vi "test Next Frame Check.vi"(8 "error in (no error)":errorcluster, 11 "BC Major Frame in":refnum<class "BC Major Frame.lvclass">) -> (0 "error out":errorcluster, 3 "BC Major Frame out":refnum<class "BC Major Frame.lvclass">)   [LabVIEW 2016, in "BC Major Frame.lvclass"]
uses:
  BC Major Frame.lvclass
  Frames & Messages/TypeDefs/BC Condition Codes.ctl
  Frames & Messages/TypeDefs/BC Op Codes - Verbose.ctl
  PPLs/FPGA Interface.lvlibp/FPGA Interface/FPGA Interface.lvclass
  BCI-1553 API.lvlib
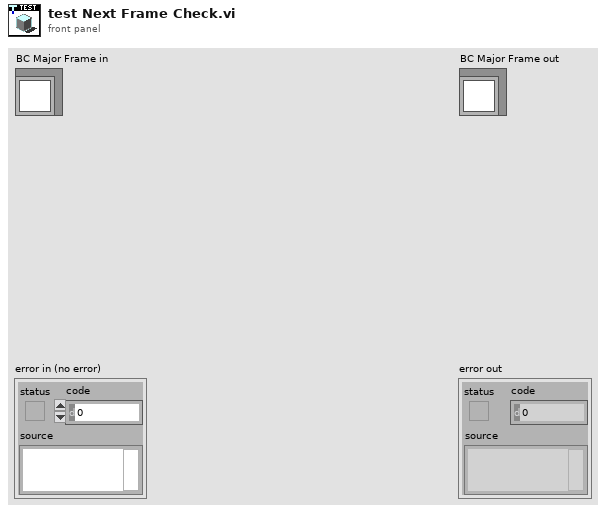
[diagram p1: front panel]
types:
  T1 = typedef "BCI-1553 API.lvlib/BC Op Codes - Verbose.ctl" = enum16{"EXECUTE MSG", "EXECUTE MSG GO", "JUMP", "CALL SUBROUTINE", "RETURN", "INTERRUPT REQUEST", "HALT", "DELAY", "WAIT FRAME TIMER = 0", "COMPARE FRAME TIMER", "COMPARE MSG TIMER", "LOAD TIME TAG CTR", "LOAD TIME TAG CTR HI", "LOAD FRAME TIMER", "START FRAME TIMER", "PUSH TIME TAG COUNT", "PUSH TIME TAG COUNT HI", "PUSH TIME TAG COUNT BOTH", "PUSH BLOCK STATUS WORD", "PUSH CURRENT VALUE", "PUSH INDIRECT", "WAIT EXT TRIGGER", "EXECUTE AND FLIP", "EXECUTE, FLIP, GO", "WRITE VALUE TO WMI", "WRITE VALUE TO MEM", "DECREMENT RAM, SKIP", "FLAG"}
  T2 = typedef "BCI-1553 API.lvlib/BC Condition Codes.ctl" = enum16{"GP0 == 1 || LT", "GP1 == 1 || NE", "GP2 == 1", "GP3 == 1", "GP4 == 1", "GP5 == 1", "GP6 == 1", "GP7 == 1", "NORESP", "FMTERR", "GOODBLOCK", "MSKSTATSET", "BADMSG", "1RETRY", "2RETRY", "ALWAYS"}
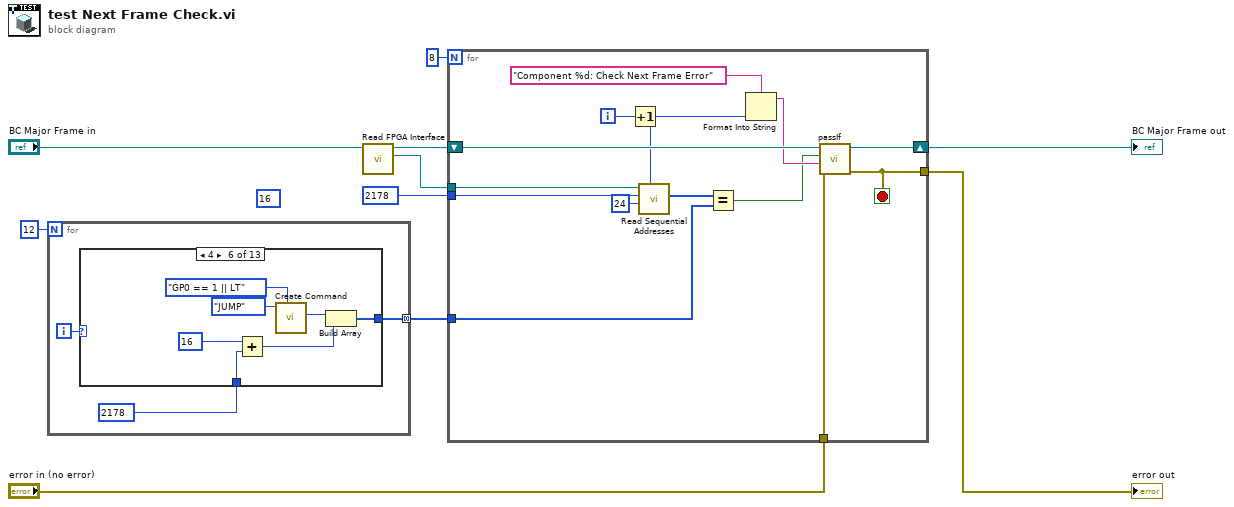
[diagram p0: block diagram]
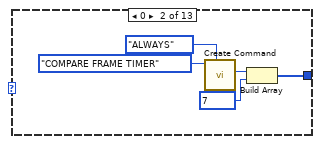
[diagram p3: hidden frame]
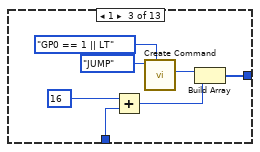
[diagram p4: hidden frame]
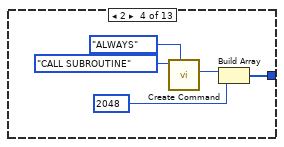
[diagram p5: hidden frame]
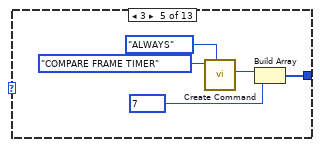
[diagram p6: hidden frame]
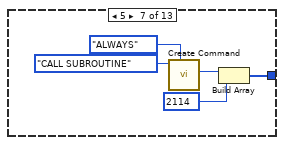
[diagram p7: hidden frame]
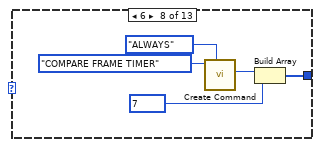
[diagram p8: hidden frame]
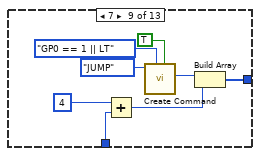
[diagram p9: hidden frame]
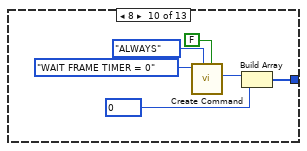
[diagram p10: hidden frame]
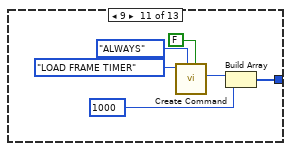
[diagram p11: hidden frame]
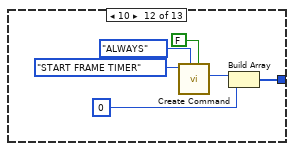
[diagram p12: hidden frame]
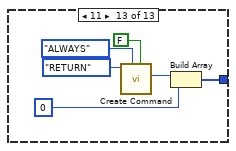
[diagram p13: hidden frame]
diagram:
  (unwired) u16 16 ("element")
  n1 = for {
    N: 12 -> [_]
    tunnel: [w12] -> w1 mode=concatenating
    i -> [w13]
    n2 = case shown="4" w13 {
      tunnel: [_ w15 w22 w27 w32 w39 w44 w49 w57 w63 w69 w75 w81] -> w12
      tunnel: u16 2178 -> [_ _ w19 _ _ w36 _ _ w53 _ _ _ _]
      frame Default {
      }
      frame 0 {
        n3 = call "Create Command.vi"("Condition"=BC_Condition_Codes."ALWAYS", "Op Code"=BC_Op_Codes_-_Verbose."COMPARE FRAME TIMER") -> ("Instruction"=w16:u16)  [unwired: 8 in, 1 out]
        n4 = Build Array(w16, u16 7 ("element")) -> (w15:u16[])
      }
      frame 1 {
        n5 = Add(x=u16 16 ("element"), y=w19) -> (x+y=w21:u16)
        n6 = call "Create Command.vi"("Condition"=BC_Condition_Codes."GP0 == 1 || LT", "Op Code"=BC_Op_Codes_-_Verbose."JUMP") -> ("Instruction"=w23:u16)  [unwired: 8 in, 1 out]
        n7 = Build Array(w23, w21) -> (w22:u16[])
      }
      frame 2 {
        n8 = call "Create Command.vi"("Condition"=BC_Condition_Codes."ALWAYS", "Op Code"=BC_Op_Codes_-_Verbose."CALL SUBROUTINE") -> ("Instruction"=w28:u16)  [unwired: 8 in, 1 out]
        n9 = Build Array(w28, u16 2048) -> (w27:u16[])
      }
      frame 3 {
        n10 = call "Create Command.vi"("Condition"=BC_Condition_Codes."ALWAYS", "Op Code"=BC_Op_Codes_-_Verbose."COMPARE FRAME TIMER") -> ("Instruction"=w33:u16)  [unwired: 8 in, 1 out]
        n11 = Build Array(w33, u16 7) -> (w32:u16[])
      }
      frame 4 {
        n12 = Add(x=u16 16 ("element"), y=w36) -> (x+y=w37:u16)
        n13 = call "Create Command.vi"("Condition"=BC_Condition_Codes."GP0 == 1 || LT", "Op Code"=BC_Op_Codes_-_Verbose."JUMP") -> ("Instruction"=w40:u16)  [unwired: 8 in, 1 out]
        n14 = Build Array(w40, w37) -> (w39:u16[])
      }
      frame 5 {
        n15 = call "Create Command.vi"("Condition"=BC_Condition_Codes."ALWAYS", "Op Code"=BC_Op_Codes_-_Verbose."CALL SUBROUTINE") -> ("Instruction"=w45:u16)  [unwired: 8 in, 1 out]
        n16 = Build Array(w45, u16 2114) -> (w44:u16[])
      }
      frame 6 {
        n17 = call "Create Command.vi"("Condition"=BC_Condition_Codes."ALWAYS", "Op Code"=BC_Op_Codes_-_Verbose."COMPARE FRAME TIMER") -> ("Instruction"=w50:u16)  [unwired: 8 in, 1 out]
        n18 = Build Array(w50, u16 7) -> (w49:u16[])
      }
      frame 7 {
        n19 = Add(x=u16 4 ("element"), y=w53) -> (x+y=w55:u16)
        n20 = call "Create Command.vi"("Invert Condition (F)"=TRUE, "Condition"=BC_Condition_Codes."GP0 == 1 || LT", "Op Code"=BC_Op_Codes_-_Verbose."JUMP") -> ("Instruction"=w58:u16)  [unwired: 7 in, 1 out]
        n21 = Build Array(w58, w55) -> (w57:u16[])
      }
      frame 8 {
        n22 = call "Create Command.vi"("Invert Condition (F)"=FALSE, "Condition"=BC_Condition_Codes."ALWAYS", "Op Code"=BC_Op_Codes_-_Verbose."WAIT FRAME TIMER = 0") -> ("Instruction"=w64:u16)  [unwired: 7 in, 1 out]
        n23 = Build Array(w64, u16 0) -> (w63:u16[])
      }
      frame 9 {
        n24 = call "Create Command.vi"("Invert Condition (F)"=FALSE, "Condition"=BC_Condition_Codes."ALWAYS", "Op Code"=BC_Op_Codes_-_Verbose."LOAD FRAME TIMER") -> ("Instruction"=w70:u16)  [unwired: 7 in, 1 out]
        n25 = Build Array(w70, u16 1000) -> (w69:u16[])
      }
      frame 10 {
        n26 = call "Create Command.vi"("Invert Condition (F)"=FALSE, "Condition"=BC_Condition_Codes."ALWAYS", "Op Code"=BC_Op_Codes_-_Verbose."START FRAME TIMER") -> ("Instruction"=w76:u16)  [unwired: 7 in, 1 out]
        n27 = Build Array(w76, u16 0) -> (w75:u16[])
      }
      frame 11 {
        n28 = call "Create Command.vi"("Invert Condition (F)"=FALSE, "Condition"=BC_Condition_Codes."ALWAYS", "Op Code"=BC_Op_Codes_-_Verbose."RETURN") -> ("Instruction"=w82:u16)  [unwired: 7 in, 1 out]
        n29 = Build Array(w82, u16 0) -> (w81:u16[])
      }
    }
  }
  n30 = call-dynamic "Read FPGA Interface.vi"("1553 Test in"="BC Major Frame in") -> ("FPGA Interface"=w9:refnum<class "FPGA Interface.lvclass">, "1553 Test out"=w10:refnum<class "BC Major Frame.lvclass">)  [unwired: 8 in, 1 out]
  n31 = for {
    N: 8 -> [_]
    shift-right: [w98] -> w5
    shift-left: w10 -> [w97]
    tunnel: w9 -> [w96]
    tunnel: u16 2178 -> [w92]
    tunnel: "error in (no error)" -> [w87]
    tunnel: [w86] -> w3
    tunnel: w1 -> [w85]
    i -> [w94]
    stop <- w86 stop-if-true
    n32 = Increment(x=w94) -> (x+1=w90:i32)
    n33 = call-dynamic "Read Sequential Addresses.vi"("Target IC (1-8)"=w90, "Addresses to Read"=u16 24, "Starting Address"=w92, "FPGA Interface in"=w96) -> ("Data"=w89:u16[])  [unwired: 6 in, 1 out]
    n34 = Equal?(x=w89, y=w85) -> (x = y?=w88:bool)
    n35 = Format Into String(format string="Component %d: Check Next Frame Error" ("custom report message (\"\")"), w90) -> (resulting string=w93:string)  [unwired: 2 in, 1 out]
    n36 = call-dynamic "passIf.vi"("error in (no error)"=w87, "message (\"\")"=w93, "pass"=w88, "TestCase in"=w97) -> ("error out"=w86:errorcluster, "TestCase out"=w98:refnum<class "BC Major Frame.lvclass">)  [unwired: 6 in]
  }
  "error out" <- w3
  "BC Major Frame out" <- w5
